vi "Get_Output.vi"(8 "error in (no error)":errorcluster, 11 "CNN in":refnum<class "CNN.lvclass">) -> (0 "error out":errorcluster, 1 "AvePC":dbl, 2 "PC Currents":dbl[](array[numeric]), 3 "CNN out":refnum<class "CNN.lvclass">)   [LabVIEW 2016, in "CNN.lvclass"]
uses:
  CNN.lvclass
  CNN.lvclass/CNN.ctl
  biCNN/Controls/Type of Neuron.ctl
panel:
  out "No PC":i32
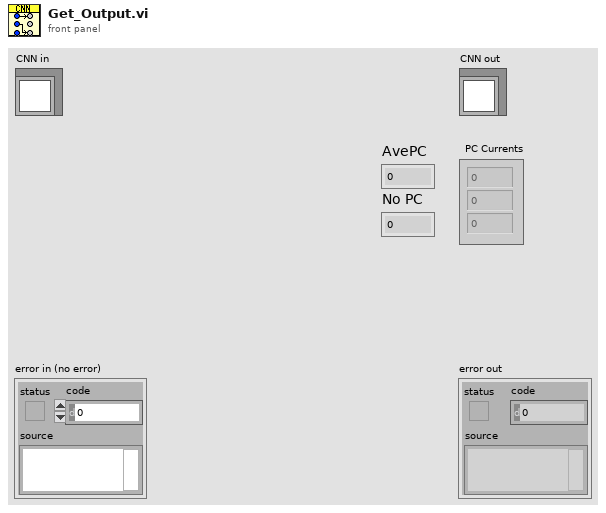
[diagram p1: front panel]
types:
  T1 = typedef "Type of Neuron.ctl" = enum16{"MF", "BA", "GO", "GC", "PC", "LU", "Glia (Dummy)"}
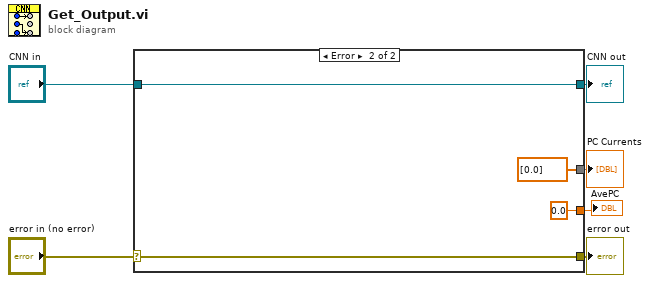
[diagram p0: block diagram]
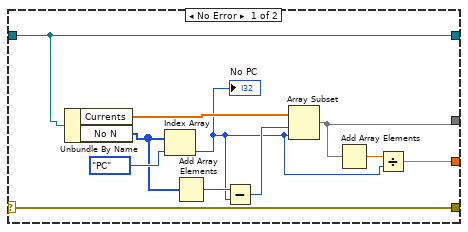
[diagram p2: hidden frame]
diagram:
  n1 = case shown="Error" "error in (no error)" {
    selector: "error in (no error)" -> [w17 w20]
    tunnel: [w17 w20] -> w5
    tunnel: [w9 w21] -> w3
    tunnel: "CNN in" -> [w9 w21]
    tunnel: [w8 dbl[] [0.0]] -> w2
    tunnel: [w7 0.0] -> w1
    frame No Error {
      n2 = Unbundle By Name(w9) -> ("Currents"=w16:dbl[], "No N"=w14:i32[])
      n3 = Index Array(array=w14, index=Type_of_Neuron."PC" ("Type of Neuron")) -> (element=w10:i32)
      "No PC" <- w10
      n4 = Add Array Elements(numeric array=w14) -> (sum=w13:i32)
      n5 = Subtract(x=w13, y=w10) -> (x-y=w12:i32)
      n6 = Array Subset(array=w16, index=w12, length=w10) -> (w8:dbl[])
      n7 = Add Array Elements(numeric array=w8) -> (sum=w11:dbl)
      n8 = Divide(x=w11, y=w10) -> (x/y=w7:dbl)
    }
    frame Error {
    }
  }
  "error out" <- w5
  "CNN out" <- w3
  "PC Currents" <- w2
  "AvePC" <- w1
